vi "teacherMain.vi"() -> ()   [LabVIEW 2022 SP3]
uses:
  teacherStates.ctl
  teacherData.ctl
  timer/timer action.ctl
panel:
  in  "Start Test":bool
  in  "Start Learning":bool
  in  "Exit":bool
  in  "Stop":bool
  in  "Polish":string
  in  "English":string
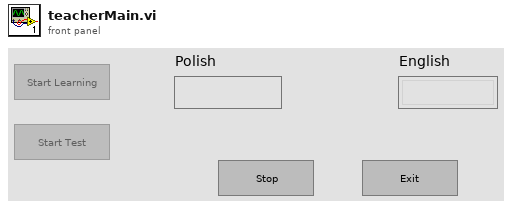
[diagram p1: front panel]
types:
  T1 = typedef "teacherStates.ctl" = enum16{"Initialize", "Idle", "LearnShowPolish", "LearnShowEnglish", "LearnReset", "TestShowPolish", "TestCheck", "Exit"}
  T2 = enum8{"Enabled", "Disabled", "Disabled and Grayed Out"}
  T3 = typedef "timer action.ctl" = enum16{"Get Time", "Reset"}
  T4 = typedef "teacherData.ctl" = cluster{"Words":string[][], "CurrentIndex":i32, "WaitTime":dbl, "NextTargetState":T1}
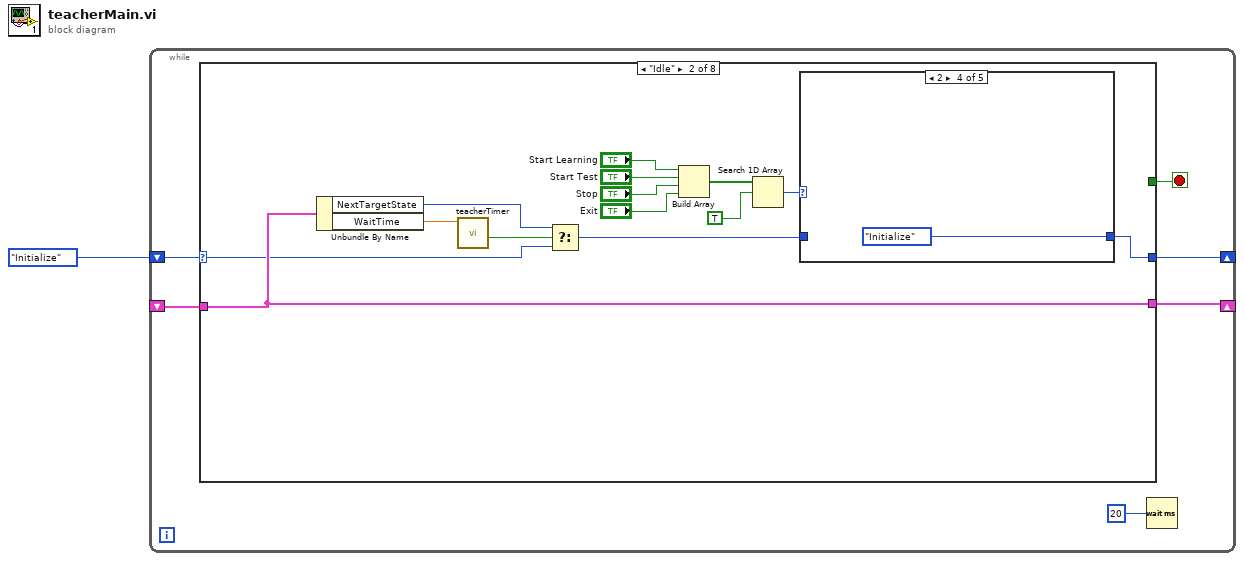
[diagram p0: block diagram]
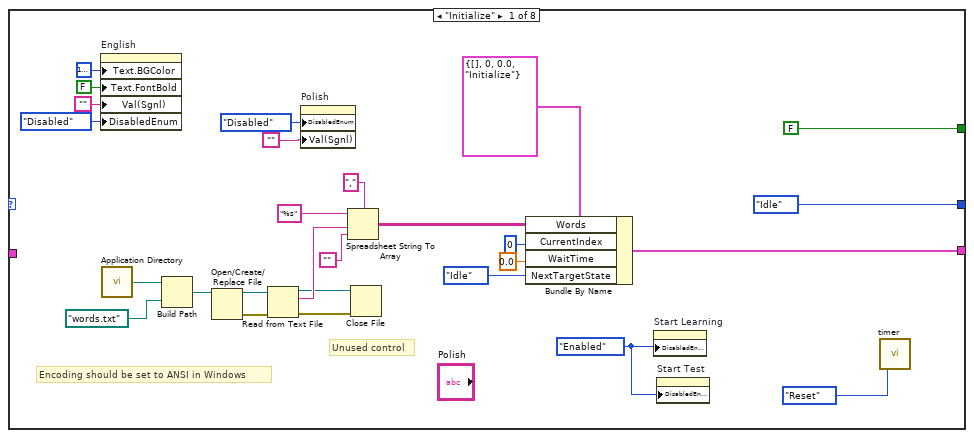
[diagram p2: hidden frame]
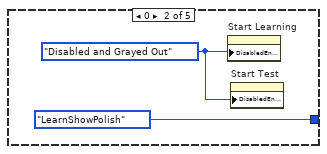
[diagram p4: hidden frame]
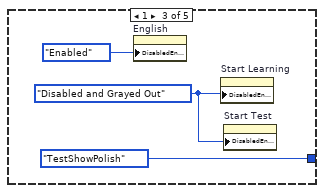
[diagram p5: hidden frame]
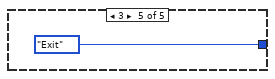
[diagram p6: hidden frame]
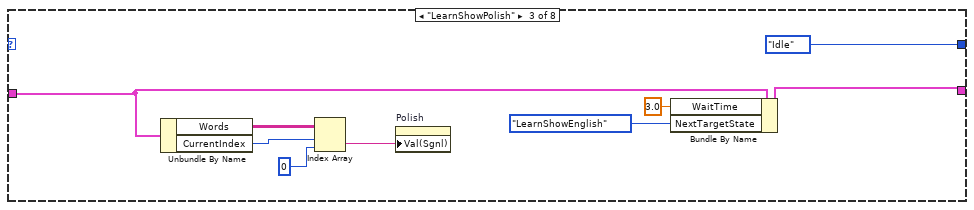
[diagram p7: hidden frame]
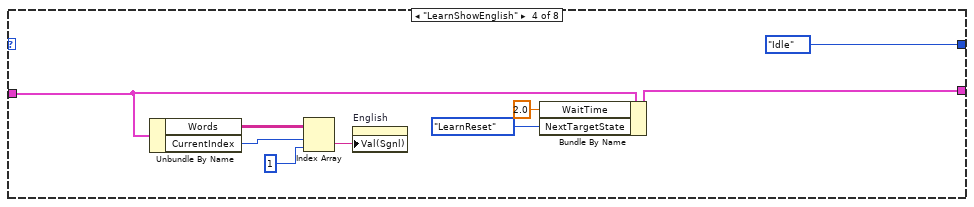
[diagram p8: hidden frame]
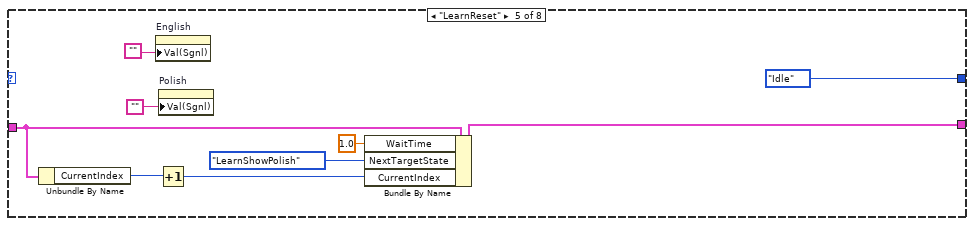
[diagram p9: hidden frame]
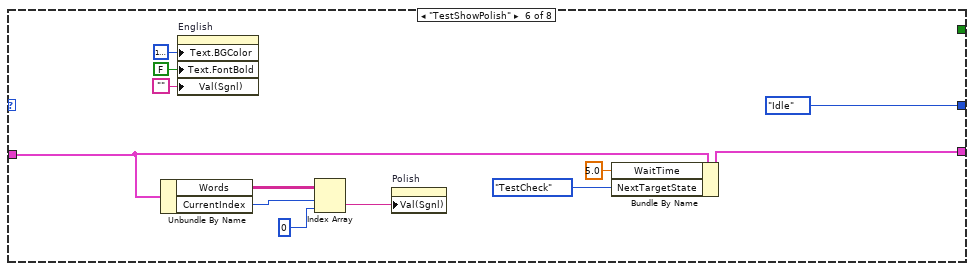
[diagram p10: hidden frame]
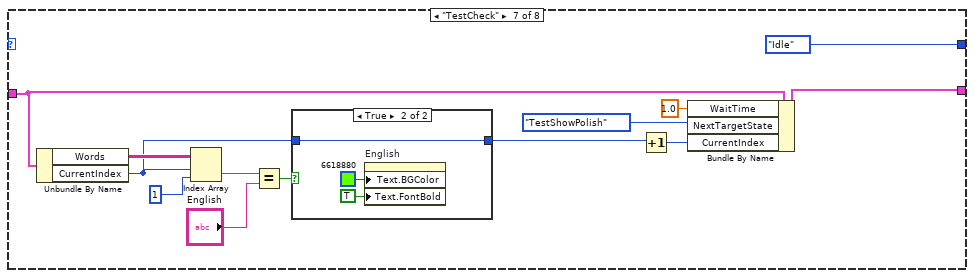
[diagram p11: hidden frame]
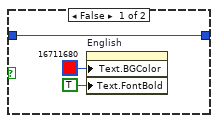
[diagram p12: hidden frame]
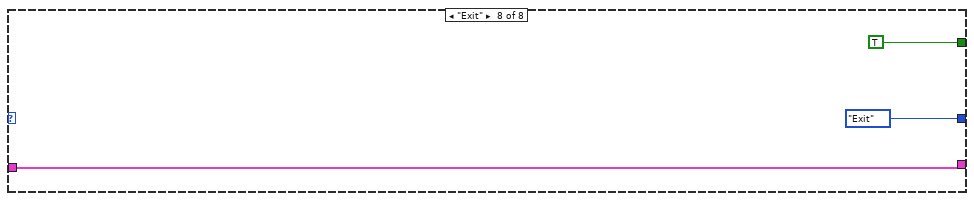
[diagram p13: hidden frame]
diagram:
  n1 = while {
    shift-right: [w3] -> _
    shift-left: teacherStates."Initialize" ("States") -> [w2]
    shift-right: [w7] -> _
    shift-left: _ -> [w5]
    stop <- w6 stop-if-true
    n2 = case shown="\"Idle\"" w2 {
      selector: w2 -> [_ w38 _ _ _ _ _ _]
      tunnel: [w20 w40 w59 w68 w78 w89 w103 w115] -> w7
      tunnel: [teacherStates."Idle" ("States") w41 teacherStates."Idle" ("States") teacherStates."Idle" ("States") teacherStates."Idle" ("States") teacherStates."Idle" ("States") teacherStates."Idle" ("States") teacherStates."Exit" ("States")] -> w3
      tunnel: [FALSE _ _ _ _ _ _ TRUE] -> w6
      tunnel: w5 -> [_ w40 w65 w74 w80 w95 w108 w115]
      frame "Initialize" {
        w8 = T2."Enabled" ("Disabled")
        # "Encoding should be set to ANSI in Windows"
        # "Unused control"
        n3 = property on="English" class="Str"("Text.BGColor"=u32 16777225 ("Text.Text Colors:BG Color"), "Text.FontBold"=FALSE ("Text.Font:Bold"), "Val(Sgnl)"="", "DisabledEnum"=T2."Disabled" ("Disabled")) -> ()  [unwired: 2 in, 2 out]
        n4 = call <vilib>:"Application Directory.vi"() -> ("Application Directory"=w32:path)
        n5 = Build Path(base path=w32, name or relative path=path "words.txt") -> (appended path=w33:path)
        n6 = Open/Create/Replace File(file path (use dialog)=w33) -> (refnum out=w28:refnum<file>, error out=w31:errorcluster)  [unwired: 5 in, 1 out]
        n7 = Read from Text File(file (use dialog)=w28, error in=w31) -> (refnum out=w29:refnum<file>, text=w34:string, error out=w30:errorcluster)  [unwired: 2 in, 1 out]
        n8 = property on="Polish" class="Str"("DisabledEnum"=T2."Disabled" ("Disabled"), "Val(Sgnl)"="") -> ()  [unwired: 2 in, 2 out]
        n9 = Spreadsheet String To Array(delimiter (Tab)=",", format string="%s", spreadsheet string=w34, array type (2D Dbl)="") -> (array=w19:string[][])
        n10 = Close File(refnum=w29, error in=w30) -> ()  [unwired: 2 out]
        n11 = Bundle By Name(cluster=T4 {"Words"=[], "CurrentIndex"=0, "WaitTime"=0.0, "NextTargetState"=enum."Initialize"} ("teacherData"), "Words"=w19, "CurrentIndex"=0 ("CurrentWord"), "WaitTime"=0.0, "NextTargetState"=teacherStates."Idle") -> (w20:T4)
        n12 = property on="Start Learning" class="Bool"("DisabledEnum"=w8) -> ()  [unwired: 2 in, 2 out]
        n13 = property on="Start Test" class="Bool"("DisabledEnum"=w8) -> ()  [unwired: 2 in, 2 out]
        n14 = call "timer.vi"("Timer action (Get Time)"=timer_action."Reset") -> ()  [unwired: 8 in, 3 out]
      }
      frame "Idle" {
        n15 = Unbundle By Name(w40) -> ("NextTargetState"=w39:T1, "WaitTime"=w36:dbl)
        n16 = call "teacherTimer.vi"("Time to elapse"=w36) -> ("Time elapsed"=w35:bool)  [unwired: 8 in, 2 out]
        n17 = Select(t=w39, s=w35, f=w38) -> (s? t:f=w37:T1)
        n18 = Build Array("Start Learning", "Start Test", "Stop", "Exit") -> (w44:bool[])
        n19 = Search 1D Array(1D array=w44, element=TRUE) -> (index of element=w42:i32)  [unwired: 1 in]
        n20 = case shown="2" w42 {
          tunnel: [w49 teacherStates."LearnShowPolish" ("States") teacherStates."TestShowPolish" ("States") teacherStates."Initialize" ("States") teacherStates."Exit" ("States")] -> w41
          tunnel: w37 -> [w49 _ _ _ _]
          frame -1, Default {
          }
          frame 0 {
            w50 = T2."Disabled and Grayed Out" ("Disabled")
            n21 = property on="Start Learning" class="Bool"("DisabledEnum"=w50) -> ()  [unwired: 2 in, 2 out]
            n22 = property on="Start Test" class="Bool"("DisabledEnum"=w50) -> ()  [unwired: 2 in, 2 out]
          }
          frame 1 {
            w53 = T2."Disabled and Grayed Out" ("Disabled")
            n23 = property on="English" class="Str"("DisabledEnum"=T2."Enabled" ("Disabled")) -> ()  [unwired: 2 in, 2 out]
            n24 = property on="Start Learning" class="Bool"("DisabledEnum"=w53) -> ()  [unwired: 2 in, 2 out]
            n25 = property on="Start Test" class="Bool"("DisabledEnum"=w53) -> ()  [unwired: 2 in, 2 out]
          }
          frame 2 {
          }
          frame 3 {
          }
        }
      }
      frame "LearnShowPolish" {
        n26 = Unbundle By Name(w65) -> ("Words"=w64:string[][], "CurrentIndex"=w62:i32)
        n27 = Index Array(array=w64, index (row)=w62, index (col)=0 ("disabled index (col)")) -> (element=w57:string)
        n28 = property on="Polish" class="Str"("Val(Sgnl)"=w57) -> ()  [unwired: 2 in, 2 out]
        n29 = Bundle By Name(cluster=w65, "WaitTime"=3.0, "NextTargetState"=teacherStates."LearnShowEnglish") -> (w59:T4)
      }
      frame "LearnShowEnglish" {
        n30 = Unbundle By Name(w74) -> ("Words"=w73:string[][], "CurrentIndex"=w71:i32)
        n31 = Index Array(array=w73, index (row)=w71, index (col)=1 ("disabled index (col)")) -> (element=w66:string)
        n32 = property on="English" class="Str"("Val(Sgnl)"=w66) -> ()  [unwired: 2 in, 2 out]
        n33 = Bundle By Name(cluster=w74, "WaitTime"=2.0, "NextTargetState"=teacherStates."LearnReset") -> (w68:T4)
      }
      frame "LearnReset" {
        n34 = Unbundle By Name(w80) -> ("CurrentIndex"=w79:i32)
        n35 = property on="English" class="Str"("Val(Sgnl)"="") -> ()  [unwired: 2 in, 2 out]
        n36 = Increment(x=w79) -> (x+1=w77:i32)
        n37 = property on="Polish" class="Str"("Val(Sgnl)"="") -> ()  [unwired: 2 in, 2 out]
        n38 = Bundle By Name(cluster=w80, "WaitTime"=1.0, "NextTargetState"=teacherStates."LearnShowPolish", "CurrentIndex"=w77) -> (w78:T4)
      }
      frame "TestShowPolish" {
        n39 = Unbundle By Name(w95) -> ("Words"=w94:string[][], "CurrentIndex"=w92:i32)
        n40 = property on="English" class="Str"("Text.BGColor"=u32 16777225 ("Text.Text Colors:BG Color"), "Text.FontBold"=FALSE ("Text.Font:Bold"), "Val(Sgnl)"="") -> ()  [unwired: 2 in, 2 out]
        n41 = Index Array(array=w94, index (row)=w92, index (col)=0 ("disabled index (col)")) -> (element=w84:string)
        n42 = property on="Polish" class="Str"("Val(Sgnl)"=w84) -> ()  [unwired: 2 in, 2 out]
        n43 = Bundle By Name(cluster=w95, "WaitTime"=5.0, "NextTargetState"=teacherStates."TestCheck") -> (w89:T4)
      }
      frame "TestCheck" {
        n44 = Unbundle By Name(w108) -> ("Words"=w107:string[][], "CurrentIndex"=w97:i32)
        n45 = Index Array(array=w107, index (row)=w97, index (col)=1 ("disabled index (col)")) -> (element=w100:string)
        n46 = Equal?(x=w100, y="English") -> (x = y?=w99:bool)
        n47 = case shown="True" w99 {
          tunnel: w97 -> [w109 w112]
          tunnel: [w109 w112] -> w96
          frame False {
            n48 = property on="English" class="Str"("Text.BGColor"=u32 16711680 ("Text.Text Colors:BG Color"), "Text.FontBold"=TRUE ("Text.Font:Bold")) -> ()  [unwired: 2 in, 2 out]
          }
          frame True {
            n49 = property on="English" class="Str"("Text.BGColor"=u32 6618880 ("Text.Text Colors:BG Color"), "Text.FontBold"=TRUE ("Text.Font:Bold")) -> ()  [unwired: 2 in, 2 out]
          }
        }
        n50 = Increment(x=w96) -> (x+1=w98:i32)
        n51 = Bundle By Name(cluster=w108, "WaitTime"=1.0, "NextTargetState"=teacherStates."TestShowPolish", "CurrentIndex"=w98) -> (w103:T4)
      }
      frame "Exit" {
      }
    }
    n52 = Wait (ms)(milliseconds to wait=u32 20) -> ()  [unwired: 1 out]
  }
